vi "Msg.vi"(7 "Actor in":refnum<class "Actor.lvclass">, 11 "Terminate Msg in":refnum<class "Terminate Msg.lvclass">) -> (0 "Error out":errorcluster, 5 "Actor out":refnum<class "Actor.lvclass">)   [LabVIEW 2025, in "jettl.lvlib" / "Terminate Msg.lvlib" / "Terminate Msg.lvclass"]
uses:
  Terminate Msg.lvclass
  Terminate Msg.lvclass/Terminate Msg.ctl
  Terminate/Terminate.lvclass
  Actor/Actor/Actor.lvclass
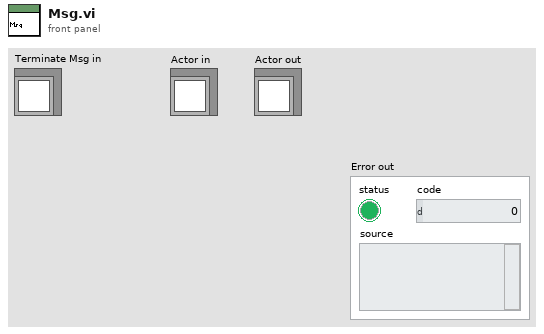
[diagram p1: front panel]
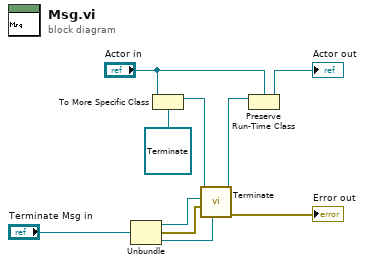
[diagram p0: block diagram]
diagram:
  n1 = Unbundle "Unbundle"("Terminate Msg in") -> (w3:refnum<class "Actor.lvclass">, w2:errorcluster, w1:refnum<class "Teller.lvclass">)
  n2 = To More Specific Class(target class=refnum<class "Terminate.lvclass"> refnum ("jettl.lvlib:jettl Msg Last Ack Creator Queue.lvlib:jettl Msg Last Ack Creator Queue.lvclass"), reference="Actor in") -> (specific class reference=w6:refnum<class "Terminate.lvclass">)  [unwired: 1 in, 1 out]
  n3 = call-dynamic "Terminate.vi"("Teller"=w1, "Error"=w2, "Actor"=w3, "Terminate in"=w6) -> ("Error out"=→"Error out":errorcluster, "Terminate out"=w5:refnum<class "Terminate.lvclass">)  [unwired: 6 in]
  n4 = Preserve Run-Time Class(object in=w5, 2:"Actor in") -> (object out=→"Actor out":refnum<class "Actor.lvclass">)  [unwired: 1 in, 1 out]
